vi "Configure Digital Line.vi"(7 "Line Direction (0: In)":i32(ring) items=["In", "Out", "Opendrain", "Master", "Acceptor"], 8 "error in (no error)":errorcluster, 9 "Line Number (1: line1)":i32(ring)=1 items=["line1"=1, "line2"=2, "line3"=3, "line4"=4, "line5"=5, "line6"=6], 10 "Line Type (0: Digital)":i32(ring) items=["Digital", "Trigger", "Synchronous"], 11 "VISA resource name":refnum<visa-resource-name>) -> (0 "error out":errorcluster, 3 "VISA resource name out":refnum<visa-resource-name>)   [LabVIEW 2016, in "Keithley DMM6500 DAQ6500 Series.lvlib"]
doc: "Sets the mode of the digital I/O line to be a digital line, trigger line, or synchronous line and sets the line to be input, output, or open-drain."
uses:
  Keithley DMM6500 DAQ6500 Series.lvlib
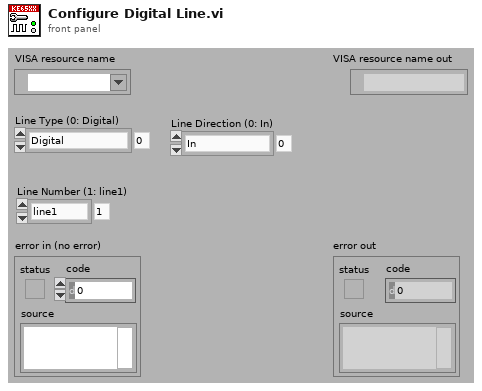
[diagram p1: front panel]
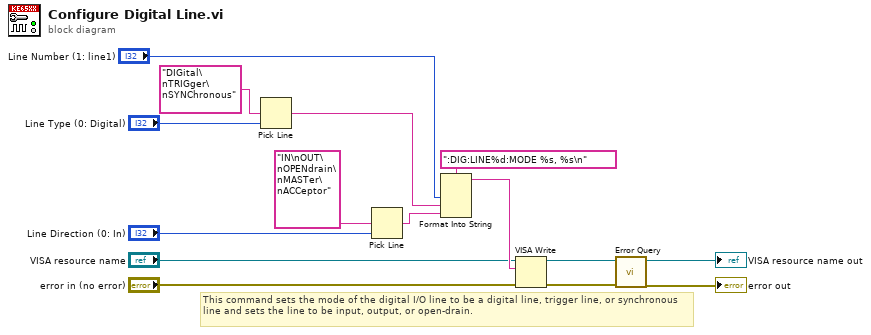
[diagram p0: block diagram]
diagram:
  # "This command sets the mode of the digital I/O line to be a digital line, trigger line, or synchronous line and sets the line to be input, output, or open-drain."
  n1 = Pick Line(multi-line string="DIGital\nTRIGger\nSYNChronous", line index="Line Type (0: Digital)") -> (output string=w2:string)  [unwired: 1 in]
  n2 = Pick Line(multi-line string="IN\nOUT\nOPENdrain\nMASTer\nACCeptor", line index="Line Direction (0: In)") -> (output string=w3:string)  [unwired: 1 in]
  n3 = Format Into String(format string=":DIG:LINE%d:MODE %s, %s\n", "Line Number (1: line1)", w2, w3) -> (resulting string=w14:string)  [unwired: 2 in, 1 out]
  n4 = VISA Write(VISA resource name="VISA resource name", write buffer=w14, error in (no error)="error in (no error)") -> (VISA resource name out=w11:refnum<visa-resource-name>, error out=w10:errorcluster)  [unwired: 1 out]
  n5 = call "Error Query.vi"("error in (no error)"=w10, "VISA resource name"=w11) -> ("error out"=→"error out":errorcluster, "VISA resource name out"=→"VISA resource name out":refnum<visa-resource-name>)  [unwired: 6 in, 2 out]
